vi "Parent Path.vi"(7 "Parent path":T1=enum."Setting", 8 "error in (no error)":errorcluster, 11 "Path in":string) -> (0 "error out":errorcluster, 3 "Path out":path)   [LabVIEW 2017, in "File.lvlib"]
uses:
  File.lvlib
  Control/Parent path.ctl
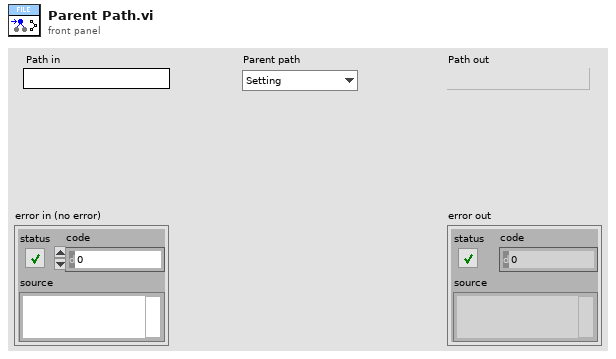
[diagram p1: front panel]
types:
  T1 = typedef "File.lvlib/Parent path.ctl" = enum16{"Project", "Setting", "Log"}
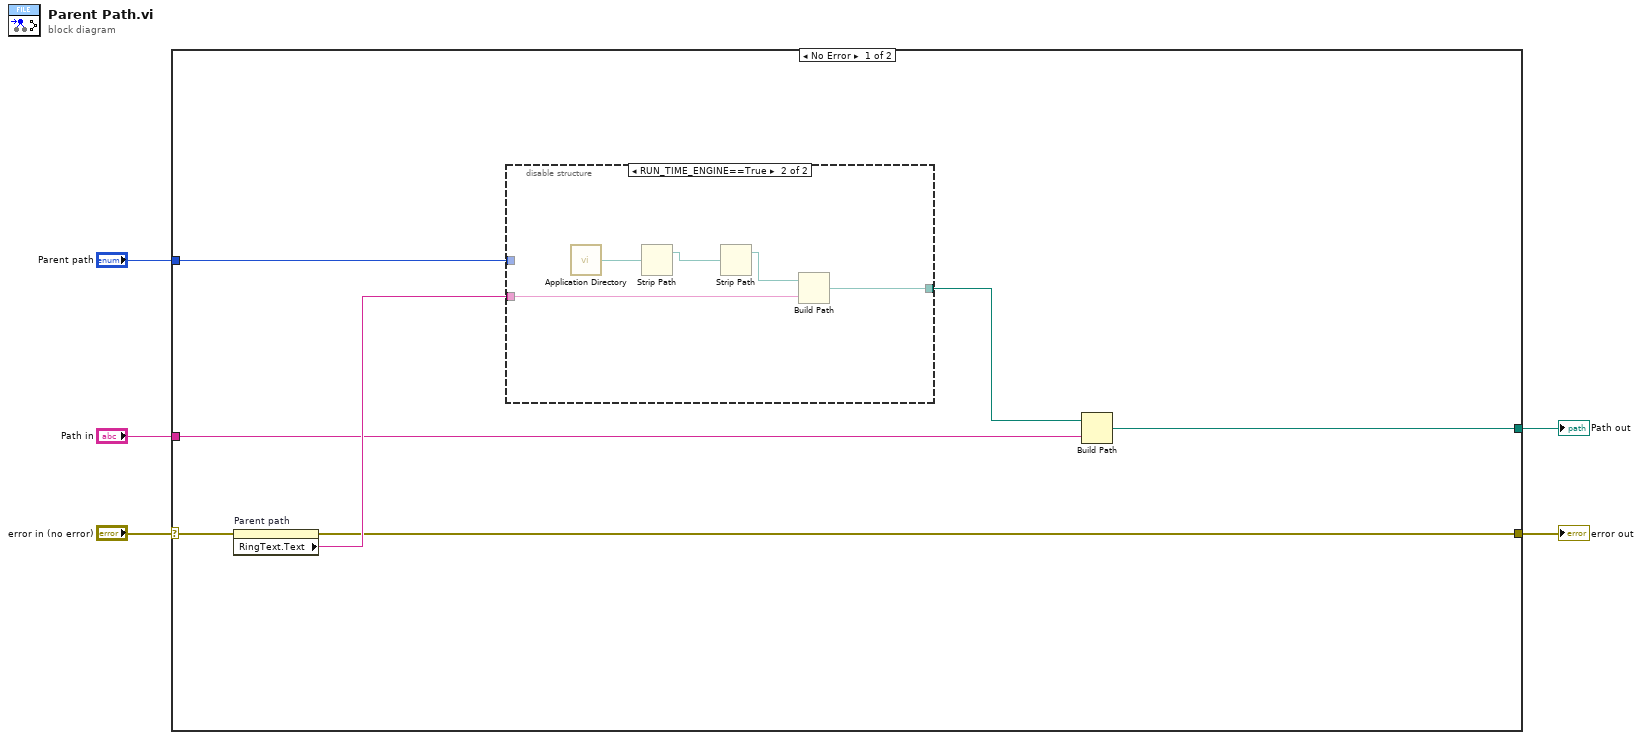
[diagram p0: block diagram]
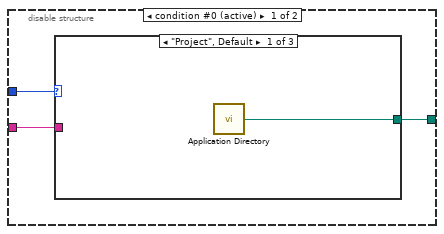
[diagram p2: hidden frame]
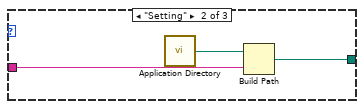
[diagram p3: hidden frame]
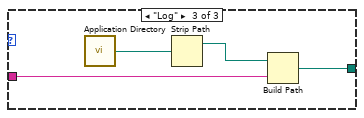
[diagram p4: hidden frame]
diagram:
  n1 = case shown="No Error" "error in (no error)" {
    selector: "error in (no error)" -> [w12 w29]
    tunnel: [w7 _] -> w3
    tunnel: [w6 w29] -> w4
    tunnel: "Path in" -> [w9 _]
    tunnel: "Parent path" -> [w11 _]
    frame No Error {
      n2 = property on="Parent path" class="Enum (strict)"(error in=w12) -> (error out=w6:errorcluster, "RingText.Text"=w10:string)  [unwired: 1 in, 1 out]
      n3 = disable-structure shown="RUN_TIME_ENGINE==True" {
        disable-tunnel: w11 -> [w15 _]
        disable-tunnel: w10 -> [w14 w26]
        disable-tunnel: [w13 w27] -> w8
        frame condition #0 (active) {
          n4 = case shown="\"Project\", Default" w15 {
            tunnel: w14 -> [_ w18 w23]
            tunnel: [w16 w17 w20] -> w13
            frame "Project", Default {
              n5 = call <vilib>:"Application Directory.vi"() -> ("Application Directory"=w16:path)
            }
            frame "Setting" {
              n6 = call <vilib>:"Application Directory.vi"() -> ("Application Directory"=w19:path)
              n7 = Build Path(base path=w19, name or relative path=w18) -> (appended path=w17:path)
            }
            frame "Log" {
              n8 = call <vilib>:"Application Directory.vi"() -> ("Application Directory"=w22:path)
              n9 = Strip Path(path=w22) -> (stripped path=w21:path)  [unwired: 1 out]
              n10 = Build Path(base path=w21, name or relative path=w23) -> (appended path=w20:path)
            }
          }
        }
        frame condition #1 {
          n11 = call <vilib>:"Application Directory.vi"() -> ("Application Directory"=w28:path)
          n12 = Strip Path(path=w28) -> (stripped path=w25:path)  [unwired: 1 out]
          n13 = Strip Path(path=w25) -> (stripped path=w24:path)  [unwired: 1 out]
          n14 = Build Path(base path=w24, name or relative path=w26) -> (appended path=w27:path)
        }
      }
      n15 = Build Path(base path=w8, name or relative path=w9) -> (appended path=w7:path)
    }
    frame Error {
    }
  }
  "error out" <- w4
  "Path out" <- w3
